vi "Lightfield.vi"() -> ()   [LabVIEW 2018]
uses:
  <vilib>/Enthought/Python Integration Toolkit/api/Console Visibility.ctl
  Global Variables.vi
  ProgramData/Documents/Princeton Instruments/LightField/Add-in and Automation SDK/Samples/LabVIEW Automation/lightfield-automation-labview/LightField Automation.lvclass
  <vilib>/Enthought/Python Integration Toolkit/Python Integration Toolkit.lvlib
panel:
  out "Position get":i32
  in  "Filter Array 2":i32[](array[numeric])=[1, 2, 3]
  in  "Power sweep":bool
  out "File Path Cam2":path=path "C:/Users/aspit/Git/MHDLab/Test Data/2018-06-28/Proj_VaporTubes/Temp Dependence/Lightfield_200C_2_Cam2"
  in  "Cam2ExperimentName":string="TestCamera2"
  in  "Use Camera 2":bool
  in  "Cam1ExperimentName":string="TestCamera"
  out "File Path Cam1":path=path "C:/Users/aspit/Git/MHDLab/Test Data/2018-06-28/Proj_VaporTubes/Temp Dependence/Lightfield_200C_2"
  in  "stop":bool
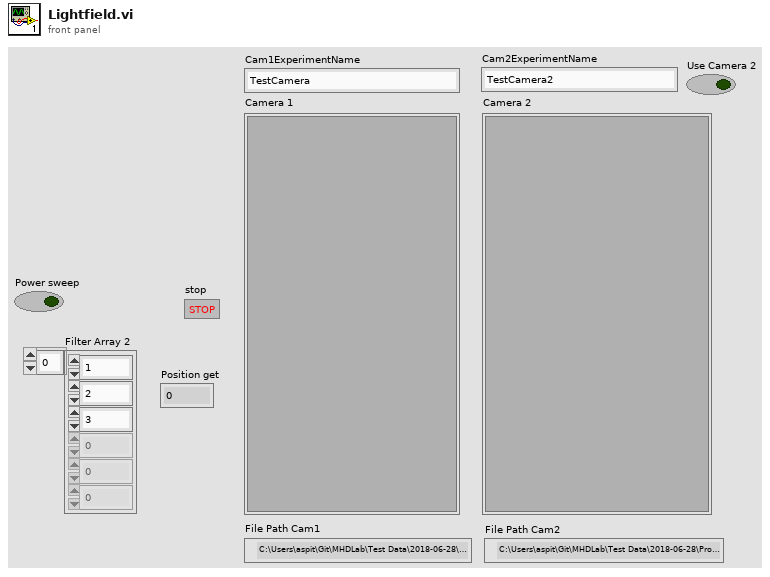
[diagram p1: front panel]
types:
  T1 = typedef "Python Integration Toolkit.lvlib/Console Visibility.ctl" = enum16{"Show Console", "Show Console While Running", "Hide Console"}
  T2 = typedef "Python Integration Toolkit.lvlib/Session ID.ctl" = u64
  T3 = typedef "Python Integration Toolkit.lvlib/Python Objects.ctl" = variant
  T4 = cluster{"Project":u16, "SubFolder":string, "Filename (Meas. Description)":string, "Measurement index":i32}
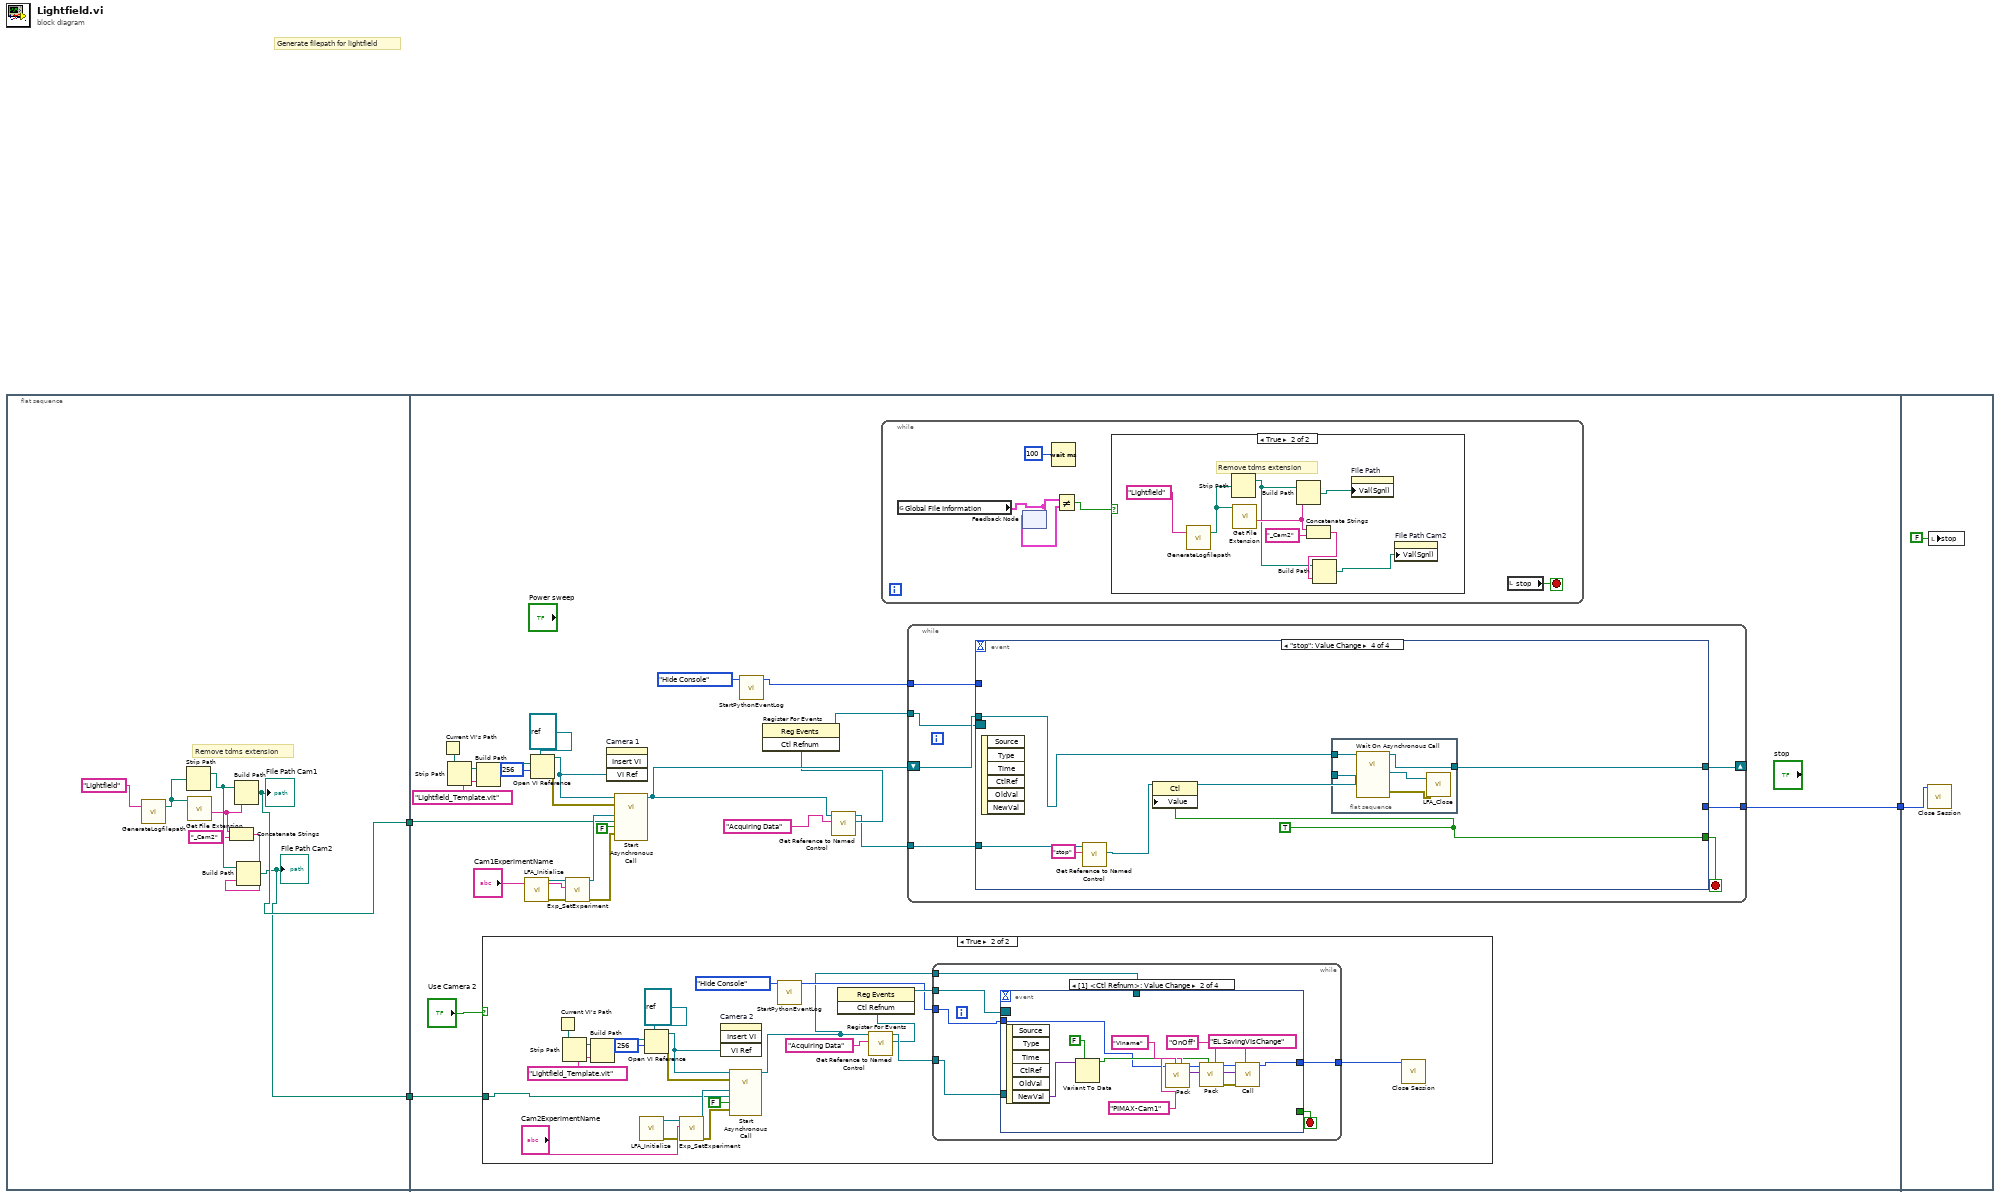
[diagram p0: block diagram]
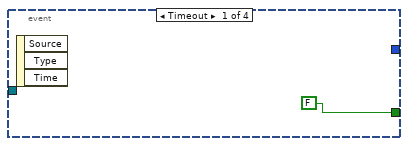
[diagram p3: hidden frame]
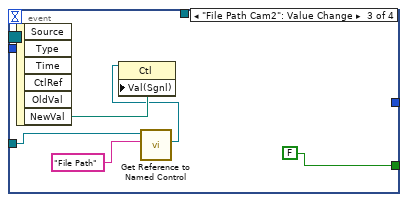
[diagram p4: hidden frame]
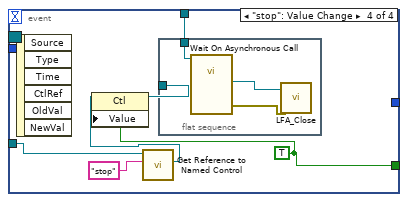
[diagram p5: hidden frame]
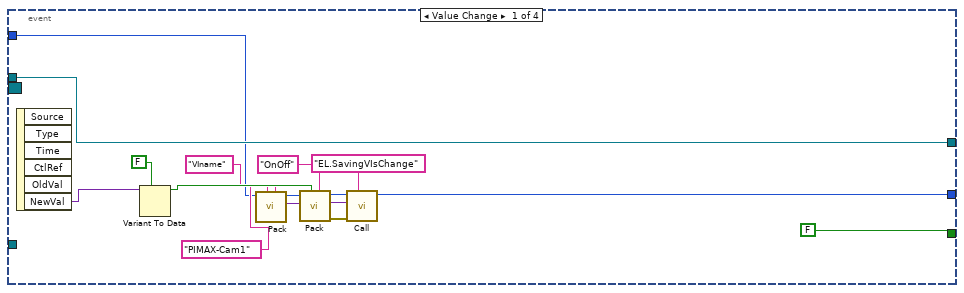
[diagram p6: hidden frame]
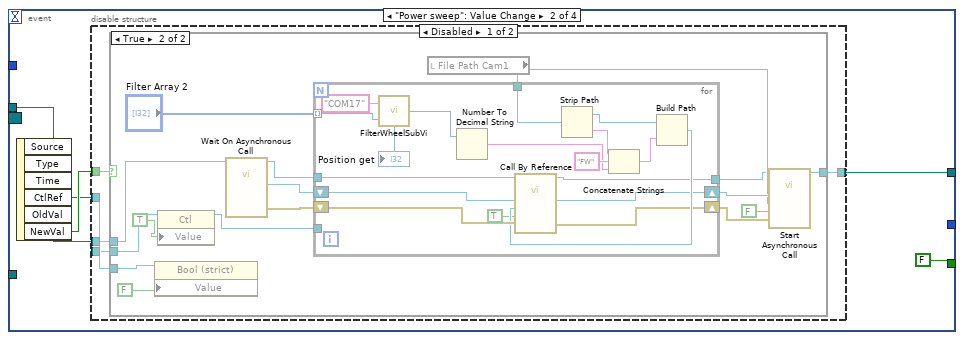
[diagram p7: hidden frame]
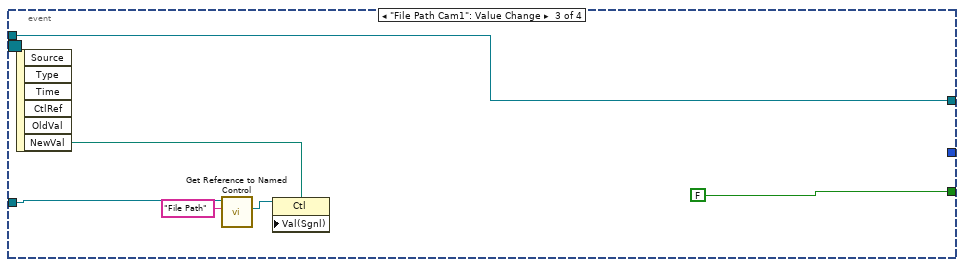
[diagram p10: hidden frame]
diagram:
  # "Generate filepath for lightfield"
  n1 = flat-sequence {
    tunnel: [w11] -> w3
    tunnel: [w10] -> w2
    tunnel: w3 -> [w23]
    tunnel: w2 -> [w22]
    tunnel: [w18] -> w1
    tunnel: w1 -> [w192]
    frame #0 {
      # "Remove tdms extension"
      n2 = call "GenerateLogfilepath.vi"("Instrument"="Lightfield") -> ("Logfile Path"=w4:path)  [unwired: 1 in, 1 out]
      n3 = Strip Path(path=w4) -> (stripped path=w8:path)  [unwired: 1 out]
      n4 = call <vilib>:"Get File Extension.vi"("file"=w4) -> ("filename without extension"=w7:string)  [unwired: 6 in, 4 out]
      n5 = Concatenate Strings(w7, "_Cam2" ("string")) -> (w5:string)
      n6 = Build Path(base path=w8, name or relative path=w7) -> (appended path=w11:path)
      "File Path Cam1" <- w11
      n7 = Build Path(base path=w8, name or relative path=w5) -> (appended path=w10:path)
      "File Path Cam2" <- w10
    }
    frame #1 {
      n8 = Current VI's Path() -> (path=w33:path)
      n9 = Strip Path(path=w33) -> (stripped path=w34:path)  [unwired: 1 out]
      n10 = Build Path(base path=w34, name or relative path="Lightfield_Template.vit") -> (appended path=w30:path)
      n11 = case shown="True" "Use Camera 2" {
        tunnel: w22 -> [_ w46]
        frame False {
        }
        frame True {
          n12 = Current VI's Path() -> (path=w50:path)
          n13 = Strip Path(path=w50) -> (stripped path=w49:path)  [unwired: 1 out]
          n14 = Build Path(base path=w49, name or relative path="Lightfield_Template.vit") -> (appended path=w53:path)
          n15 = call "LFA_Initialize.vi"() -> ("error out"=w47:errorcluster, "LightField Automation out"=w48:refnum<class "LightField Automation.lvclass">)  [unwired: 10 in]
          n16 = Open VI Reference(type specifier VI Refnum (for type only)=refnum<vi> refnum, vi path=w53, options=256) -> (vi reference=w55:refnum<vi>, error out=w56:errorcluster)  [unwired: 1 in, 2 out]
          n17 = call "Exp_SetExperiment.vi"("error in (no error)"=w47, "ExperimentName"="Cam2ExperimentName", "LightField Automation in"=w48) -> ("error out"=w57:errorcluster, "LightField Automation out"=w58:refnum<class "LightField Automation.lvclass">)  [unwired: 7 in]
          n18 = invoke on="Camera 2" class="SubPnl" method="Insert VI"("VI Ref"=w55) -> ()  [unwired: 3 in, 4 out]
          n19 = call-by-ref "Start Asynchronous Call"(reference=w55, error in=w56, "error out"=w57, "Single Run"=FALSE, "Filepath"=w46, "LightField Automation in"=w58) -> (reference out=w37:refnum<vi>)  [unwired: 6 in, 3 out]
          n20 = call "StartPythonEventLog.vi"("Console Visibility"=Console_Visibility."Hide Console") -> ("Session ID out"=w43:T2)  [unwired: 10 in]
          n21 = call "Get Reference to Named Control.vi"("Control Name"="Acquiring Data" ("element"), "Front Panel Ref"=w37) -> ("Ctl Refnum"=w39:refnum<vi>, "Panel Ref Out"=w40:refnum<vi>)  [unwired: 7 in, 1 out]
          n22 = register-events(w39) -> (reference out=w44:refnum<event-registration>)  [unwired: 2 in, 1 out]
          n23 = while {
            tunnel: w40 -> [w64]
            tunnel: w43 -> [w62]
            tunnel: w44 -> [w63]
            tunnel: [w61] -> w42
            tunnel: w37 -> [w60]
            stop <- w65 stop-if-true
            n24 = event shown="[1] <Ctl Refnum>: Value Change" {
              selector: w63 -> [_ _ _ _]
              dyn-events: _ -> [_ _ _ _]
              timeout: _ -> [_ _ _ _]
              tunnel: [FALSE _ FALSE w91] -> w65
              tunnel: w64 -> [_ _ w83 w88]
              tunnel: w62 -> [_ w68 _ _]
              tunnel: [_ w67 _ _] -> w61
              tunnel: w60 -> [_ _ _ w86]
              event Timeout {
                n25 = event-data() -> ()  [unwired: 1 in, 3 out]
              }
              event Value Change {
                n26 = event-data() -> ("NewVal"=w69:variant)  [unwired: 1 in, 5 out]
                n27 = Variant To Data(type=FALSE, Variant=w69) -> (data=w71:bool)  [unwired: 1 in, 1 out]
                n28 = call <vilib>:"Pack.vi"("Keyword Name"="VIname", "Argument"="PIMAX-Cam1", "Session ID"=w68) -> ("Python Object References Out"=w79:T3, "Session ID out"=w75:T2)  [unwired: 6 in, 1 out]
                n29 = call <vilib>:"Pack.vi"("Keyword Name"="OnOff", "Argument"=w71, "Python Object References In"=w79, "Session ID"=w75) -> ("error out"=w76:errorcluster, "Python Object References Out"=w77:T3, "Session ID out"=w78:T2)  [unwired: 5 in]
                n30 = call <vilib>:"Call.vi"("Function or Method Name"="EL.SavingVIsChange", "error in (no error)"=w76, "Python Object References In"=w77, "Session ID"=w78) -> ("Session ID out"=w67:T2)  [unwired: 5 in, 2 out]
              }
              event "File Path Cam2": Value Change {
                n31 = event-data() -> ("NewVal"=w85:path)  [unwired: 1 in, 5 out]
                n32 = call "Get Reference to Named Control.vi"("Control Name"="File Path" ("element"), "Front Panel Ref"=w83) -> ("Ctl Refnum"=w81:refnum<vi>)  [unwired: 7 in, 2 out]
                n33 = property class="Ctl"(reference=w81, "Val(Sgnl)"=w85) -> ()  [unwired: 1 in, 2 out]
              }
              event "stop": Value Change {
                w91 = TRUE
                n34 = event-data() -> ()  [unwired: 1 in, 6 out]
                n35 = call "Get Reference to Named Control.vi"("Control Name"="stop" ("element"), "Front Panel Ref"=w88) -> ("Ctl Refnum"=w87:refnum<vi>)  [unwired: 7 in, 2 out]
                n36 = property class="Ctl"(reference=w87, "Value"=w91) -> (reference out=w90:refnum<vi>)  [unwired: 1 in, 1 out]
                n37 = flat-sequence {
                  tunnel: w90 -> [_]
                  tunnel: w86 -> [w92]
                  frame #0 {
                    n38 = call-by-ref "Wait On Asynchronous Call"(reference=w92) -> ("error out 2"=w93:errorcluster, "LightField Automation out"=w94:refnum<class "LightField Automation.lvclass">)  [unwired: 11 in, 2 out]
                    n39 = call "LFA_Close.vi"("error in (no error)"=w93, "LightField Automation in"=w94) -> ()  [unwired: 8 in, 2 out]
                  }
                }
              }
            }
          }
          n40 = call <vilib>:"Close Session.vi"("Session ID"=w42) -> ()  [unwired: 10 in, 1 out]
        }
      }
      n41 = call "LFA_Initialize.vi"() -> ("error out"=w36:errorcluster, "LightField Automation out"=w35:refnum<class "LightField Automation.lvclass">)  [unwired: 10 in]
      n42 = Open VI Reference(type specifier VI Refnum (for type only)=refnum<vi> refnum, vi path=w30, options=256) -> (vi reference=w28:refnum<vi>, error out=w27:errorcluster)  [unwired: 1 in, 2 out]
      n43 = call "Exp_SetExperiment.vi"("error in (no error)"=w36, "ExperimentName"="Cam1ExperimentName", "LightField Automation in"=w35) -> ("error out"=w26:errorcluster, "LightField Automation out"=w25:refnum<class "LightField Automation.lvclass">)  [unwired: 7 in]
      n44 = invoke on="Camera 1" class="SubPnl" method="Insert VI"("VI Ref"=w28) -> ()  [unwired: 3 in, 4 out]
      n45 = call-by-ref "Start Asynchronous Call"(reference=w28, error in=w27, "error out"=w26, "Single Run"=FALSE, "Filepath"=w23, "LightField Automation in"=w25) -> (reference out=w17:refnum<vi>)  [unwired: 6 in, 3 out]
      n46 = call "StartPythonEventLog.vi"("Console Visibility"=Console_Visibility."Hide Console") -> ("Session ID out"=w19:T2)  [unwired: 10 in]
      n47 = call "Get Reference to Named Control.vi"("Control Name"="Acquiring Data" ("element"), "Front Panel Ref"=w17) -> ("Ctl Refnum"=w15:refnum<vi>, "Panel Ref Out"=w14:refnum<vi>)  [unwired: 7 in, 1 out]
      n48 = register-events(w15) -> (reference out=w20:refnum<event-registration>)  [unwired: 2 in, 1 out]
      n49 = while {
        stop <- w183 stop-if-true
        n50 = global read "Global Variables.vi" "Global File Information"() -> (w181:T4)
        n51 = feedback #1() -> (w180:T4)  [unwired: 1 in]
        n52 = feedback-in #1(w181) -> ()
        n53 = Wait (ms)(milliseconds to wait=100) -> ()  [unwired: 1 out]
        n54 = Not Equal?(x=w181, y=w180) -> (x != y?=w179:bool)
        n55 = case shown="True" w179 {
          frame False {
          }
          frame True {
            # "Remove tdms extension"
            n56 = call "GenerateLogfilepath.vi"("Instrument"="Lightfield") -> ("Logfile Path"=w184:path)  [unwired: 1 in, 1 out]
            n57 = Strip Path(path=w184) -> (stripped path=w187:path)  [unwired: 1 out]
            n58 = call <vilib>:"Get File Extension.vi"("file"=w184) -> ("filename without extension"=w188:string)  [unwired: 6 in, 4 out]
            n59 = Build Path(base path=w187, name or relative path=w188) -> (appended path=w185:path)
            n60 = Concatenate Strings(w188, "_Cam2" ("string")) -> (w190:string)
            n61 = Build Path(base path=w187, name or relative path=w190) -> (appended path=w186:path)
            n62 = property on="File Path" class="Path"("Val(Sgnl)"=w185) -> ()  [unwired: 2 in, 2 out]
            n63 = property on="File Path Cam2" class="Path"("Val(Sgnl)"=w186) -> ()  [unwired: 2 in, 2 out]
          }
        }
        n64 = local read "stop"() -> (w183:bool)
      }
      n65 = while {
        shift-right: [w99] -> _
        shift-left: w17 -> [w100]
        tunnel: w20 -> [w98]
        tunnel: w19 -> [w97]
        tunnel: [w96] -> w18
        tunnel: w14 -> [w95]
        stop <- w101 stop-if-true
        n66 = event shown="[3] \"stop\": Value Change" {
          selector: w98 -> [_ _ _ _]
          dyn-events: _ -> [_ _ _ _]
          timeout: _ -> [_ _ _ _]
          tunnel: [FALSE FALSE FALSE w174] -> w101
          tunnel: w100 -> [w116 w120 w165 w173]
          tunnel: [w116 w119 w165 w172] -> w99
          tunnel: w97 -> [w109 _ _ _]
          tunnel: [w102 _ _ _] -> w96
          tunnel: w95 -> [_ _ w163 w170]
          event Value Change {
            n67 = event-data() -> ("NewVal"=w115:variant)  [unwired: 1 in, 5 out]
            n68 = Variant To Data(type=FALSE, Variant=w115) -> (data=w113:bool)  [unwired: 1 in, 1 out]
            n69 = call <vilib>:"Pack.vi"("Keyword Name"="VIname", "Argument"="PIMAX-Cam1", "Session ID"=w109) -> ("Python Object References Out"=w104:T3, "Session ID out"=w108:T2)  [unwired: 6 in, 1 out]
            n70 = call <vilib>:"Pack.vi"("Keyword Name"="OnOff", "Argument"=w113, "Python Object References In"=w104, "Session ID"=w108) -> ("error out"=w107:errorcluster, "Python Object References Out"=w106:T3, "Session ID out"=w105:T2)  [unwired: 5 in]
            n71 = call <vilib>:"Call.vi"("Function or Method Name"="EL.SavingVIsChange", "error in (no error)"=w107, "Python Object References In"=w106, "Session ID"=w105) -> ("Session ID out"=w102:T2)  [unwired: 5 in, 2 out]
          }
          event "Power sweep": Value Change {
            n72 = event-data() -> ("CtlRef"=w118:refnum<vi>, "NewVal"=w121:bool)  [unwired: 1 in, 4 out]
            n73 = disable-structure shown="Disabled" {
              disable-tunnel: w121 -> [w127 _]
              disable-tunnel: w120 -> [w126 _]
              disable-tunnel: [w125 _] -> w119
              disable-tunnel: w118 -> [w124 _]
              disable-tunnel: _ -> [w123 _]
              frame Disabled {
                n74 = case shown="True" w127 {
                  tunnel: w126 -> [w128 w143]
                  tunnel: [w128 w135] -> w125
                  tunnel: w124 -> [_ w134]
                  tunnel: w123 -> [_ w132]
                  frame False {
                  }
                  frame True {
                    n75 = property class="Bool (strict)"(reference=w134, "Value"=FALSE) -> ()  [unwired: 1 in, 2 out]
                    n76 = property class="Ctl"(reference=w132, "Value"=TRUE) -> (reference out=w130:refnum<vi>)  [unwired: 1 in, 1 out]
                    n77 = call-by-ref "Wait On Asynchronous Call"(reference=w143) -> (reference out=w129:refnum<vi>, "error out 2"=w141:errorcluster, "LightField Automation out"=w142:refnum<class "LightField Automation.lvclass">)  [unwired: 11 in, 1 out]
                    n78 = local read "File Path Cam1"() -> (w138:path)
                    n79 = for {
                      tunnel: "Filter Array 2" -> [w147] mode=indexing
                      tunnel: w129 -> [w151]
                      shift-right: [w153] -> w140
                      shift-left: w142 -> [w161]
                      shift-right: [w152] -> w139
                      shift-left: w141 -> [w160]
                      tunnel: w138 -> [w149]
                      tunnel: [w148] -> w136
                      tunnel: w130 -> [_]
                      n80 = call "FilterWheelSubVi.vi"("Position set"=w147, "Serial Port"="COM17") -> ("Position get"=w145:i32)
                      "Position get" <- w145
                      n81 = Number To Decimal String(number=w145) -> (decimal integer string=w155:string)  [unwired: 1 in]
                      n82 = Strip Path(path=w149) -> (stripped path=w159:path, name=w157:string)
                      n83 = Concatenate Strings(w157, "FW" ("string"), w155) -> (w154:string)
                      n84 = Build Path(base path=w159, name or relative path=w154) -> (appended path=w158:path)
                      n85 = call-by-ref "?"(reference=w151, "error out"=w160, "Single Run"=TRUE, "Filepath"=w158, "LightField Automation in"=w161) -> (reference out=w148:refnum<vi>, "error out 2"=w152:errorcluster, "LightField Automation out"=w153:refnum<class "LightField Automation.lvclass">)  [unwired: 7 in, 1 out]
                    }
                    n86 = call-by-ref "Start Asynchronous Call"(reference=w136, "error out"=w139, "Single Run"=FALSE, "Filepath"=w138, "LightField Automation in"=w140) -> (reference out=w135:refnum<vi>)  [unwired: 7 in, 3 out]
                  }
                }
              }
              frame Enabled {
              }
            }
          }
          event "File Path Cam1": Value Change {
            n87 = event-data() -> ("NewVal"=w167:path)  [unwired: 1 in, 5 out]
            n88 = call "Get Reference to Named Control.vi"("Control Name"="File Path" ("element"), "Front Panel Ref"=w163) -> ("Ctl Refnum"=w162:refnum<vi>)  [unwired: 7 in, 2 out]
            n89 = property class="Ctl"(reference=w162, "Val(Sgnl)"=w167) -> ()  [unwired: 1 in, 2 out]
          }
          event "stop": Value Change {
            w174 = TRUE
            n90 = event-data() -> ()  [unwired: 1 in, 6 out]
            n91 = call "Get Reference to Named Control.vi"("Control Name"="stop", "Front Panel Ref"=w170) -> ("Ctl Refnum"=w168:refnum<vi>)  [unwired: 7 in, 2 out]
            n92 = property class="Ctl"(reference=w168, "Value"=w174) -> (reference out=w171:refnum<vi>)  [unwired: 1 in, 1 out]
            n93 = flat-sequence {
              tunnel: w173 -> [w178]
              tunnel: w171 -> [_]
              tunnel: [w175] -> w172
              frame #0 {
                n94 = call-by-ref "Wait On Asynchronous Call"(reference=w178) -> (reference out=w175:refnum<vi>, "error out 2"=w176:errorcluster, "LightField Automation out"=w177:refnum<class "LightField Automation.lvclass">)  [unwired: 11 in, 1 out]
                n95 = call "LFA_Close.vi"("error in (no error)"=w176, "LightField Automation in"=w177) -> ()  [unwired: 8 in, 2 out]
              }
            }
          }
        }
      }
    }
    frame #2 {
      n96 = call <vilib>:"Close Session.vi"("Session ID"=w192) -> ()  [unwired: 10 in, 1 out]
      n97 = local write "stop"(FALSE ("stop")) -> ()
    }
  }
